vi "Camera Selection and Snap Image.vi"() -> ()   [LabVIEW 2023]
uses:
  <vilib>/vision/driver/NI_Vision_Acquisition_Software.lvlib
panel:
  in  "No Camera/Camera Present":bool
  in  "error in":errorcluster
  out "VendorName":string[](array[string])
  out "Image Display":T1(plugin-control)
  out "Camera Information Array":T2(array[cluster]) {"BusType" format="%x"; "SerialNumberLow" format="%.0x"; "SerialNumberHigh" format="%.0x"}
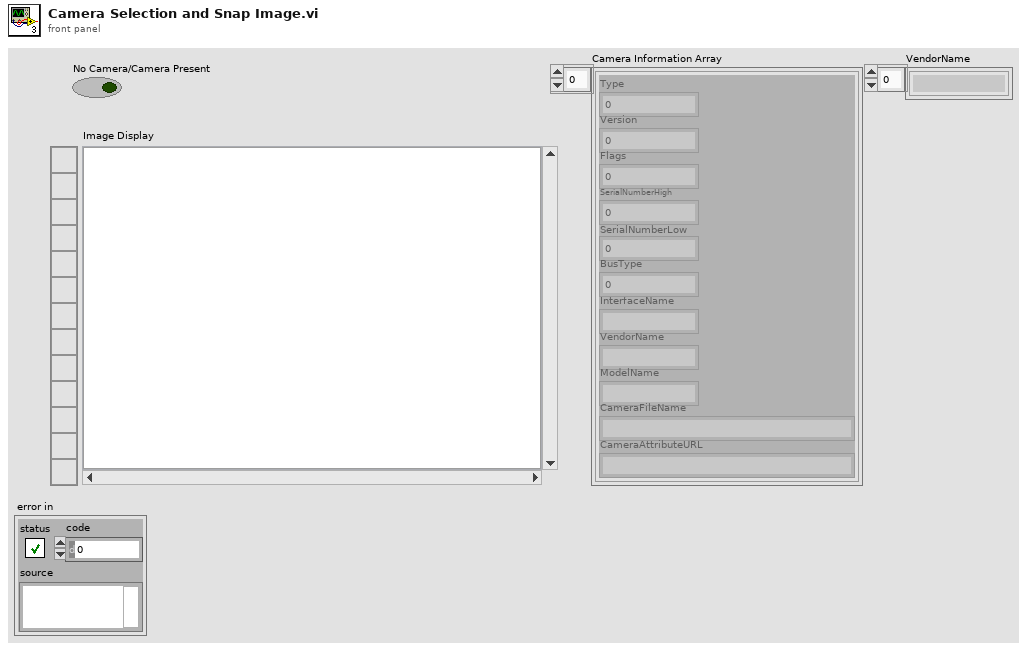
[diagram p1: front panel]
types:
  T1 = typedef "IMAQ Image.ctl" = refnum<image>
  T2 = cluster{"Type":u32, "Version":u32, "Flags":u32, "SerialNumberHigh":u32, "SerialNumberLow":u32, "BusType":u32, "InterfaceName":string, "VendorName":string, "ModelName":string, "CameraFileName":string, "CameraAttributeURL":string}[]
  T3 = typedef "IMAQdx.ctl" = refnum<k21>
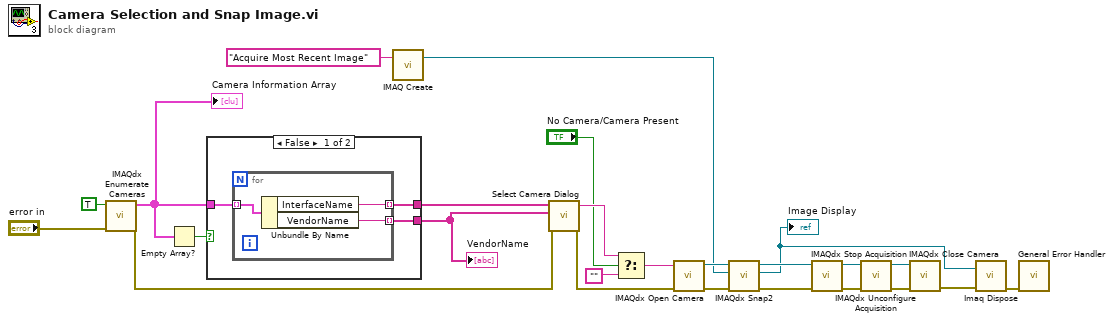
[diagram p0: block diagram]
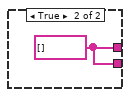
[diagram p2: hidden frame]
diagram:
  n1 = call <vilib>:"IMAQdx Enumerate Cameras.vi"("error in"="error in", "Connected Only? (Yes)"=TRUE) -> ("error out"=w6:errorcluster, "Camera Information Array"=w10:T2)  [unwired: 8 in]
  "Camera Information Array" <- w10
  n2 = Empty Array?(array=w10) -> (empty?=w11:bool)
  n3 = case shown="False" w11 {
    tunnel: w10 -> [w28 _]
    tunnel: [w27 w32] -> w8
    tunnel: [w26 w32] -> w9
    frame False {
      n4 = for {
        tunnel: w28 -> [w31] mode=indexing
        tunnel: [w30] -> w27 mode=indexing
        tunnel: [w29] -> w26 mode=indexing
        n5 = Unbundle By Name(w31) -> ("InterfaceName"=w30:string, "VendorName"=w29:string)
      }
    }
    frame True {
      w32 = string[] []
    }
  }
  "VendorName" <- w9
  n6 = call "IMAQ Create"("Image Name"="Acquire Most Recent Image") -> ("New Image"=w13:T1)  [unwired: 3 in, 2 out]
  n7 = call "Select Camera Dialog.vi"("error in (no error)"=w6, "Vendor Name"=w9, "Camera Name"=w8) -> ("error out"=w5:errorcluster, "Interface Name"=w4:string)  [unwired: 6 in, 1 out]
  n8 = Select(t=w4, s="No Camera/Camera Present", f="") -> (s? t:f=w1:string)
  n9 = call <vilib>:"IMAQdx Open Camera.vi"("error in"=w5, "Session In"=w1) -> ("error out"=w22:errorcluster, "Session Out"=w23:T3)  [unwired: 1 in, 7 out]
  n10 = call <vilib>:"IMAQdx Snap2.vi"("error in"=w22, "Image In"=w13, "Session In"=w23) -> ("error out"=w21:errorcluster, "Image Out"=w12:T1, "Session Out"=w20:T3)  [unwired: 6 in]
  "Image Display" <- w12
  n11 = call <vilib>:"IMAQdx Stop Acquisition.vi"("error in"=w21, "Session In"=w20) -> ("error out"=w16:errorcluster, "Session Out"=w17:T3)  [unwired: 8 out]
  n12 = call <vilib>:"IMAQdx Unconfigure Acquisition.vi"("error in"=w16, "Session In"=w17) -> ("error out"=w19:errorcluster, "Session Out"=w18:T3)  [unwired: 8 out]
  n13 = call <vilib>:"IMAQdx Close Camera.vi"("error in"=w19, "Session In"=w18) -> ("error out"=w15:errorcluster)  [unwired: 9 out]
  n14 = call "Imaq Dispose"("Image"=w12, "error in (no error)"=w15) -> ("error out"=w14:errorcluster)  [unwired: 4 in]
  n15 = call <vilib>:"General Error Handler.vi"("error in (no error)"=w14) -> ()  [unwired: 2 in, 13 out]
